vi "Extract Stage Status.vi"(11 "Table Stages":T4) -> (1 "Z Stage":T1, 2 "Y Stage":T1, 3 "X Stage":T1)   [LabVIEW 2018]
uses:
  Hardware Mfg/Thorlabs Translation Stages/Controls/Translation Stage Cluster.ctl
  Controls/Translation Stage Types.ctl
  Controls/Translation Stage Quick Status.ctl
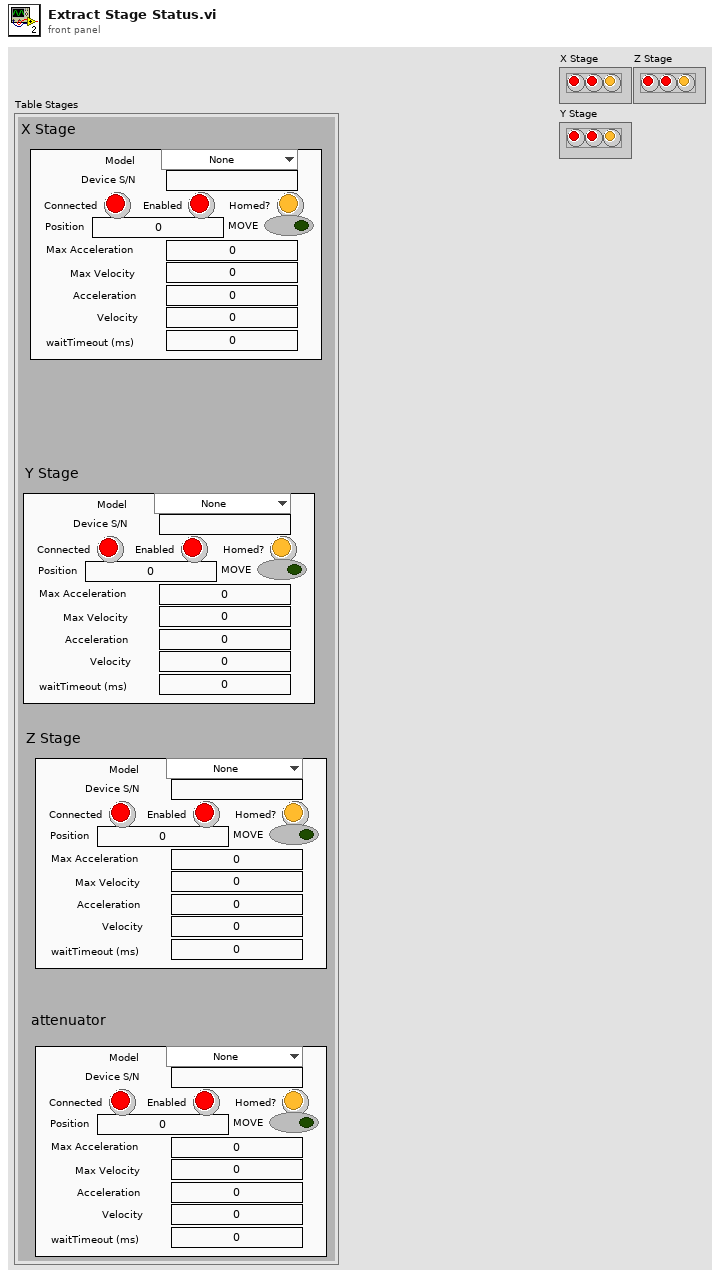
[diagram p1: front panel]
types:
  T1 = typedef "Translation Stage Quick Status.ctl" = cluster{"Is.Enabled?":bool, "Is.Connected?":bool, "Is.Homed?":bool}
  T2 = typedef "Translation Stage Cluster.ctl" = cluster{"Position":dbl, "Is.Enabled?":bool, "Is.Connected?":bool, "Device SN":string, "AccelerationMaximum":dbl, "VelocityMaximum":dbl, "Acceleration":dbl, "Velocity":dbl, "waitTimeout (ms)":i32, "Model":T3, "Is.Homed?":bool, "MOVE":bool}
  T3 = typedef "Translation Stage Types.ctl" = enum16{"None", "Thorlabs LTS", "Thorlabs MLJ"}
  T4 = cluster{"X Stage":T2, "Y Stage":T2, "Z Stage":T2, "attenuator":T2}
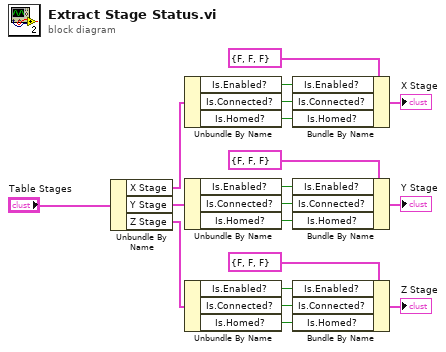
[diagram p0: block diagram]
diagram:
  n1 = Unbundle By Name("Table Stages") -> ("X Stage"=w16:T2, "Y Stage"=w15:T2, "Z Stage"=w14:T2)
  n2 = Unbundle By Name(w16) -> ("Is.Enabled?"=w9:bool, "Is.Connected?"=w8:bool, "Is.Homed?"=w7:bool)
  n3 = Unbundle By Name(w15) -> ("Is.Enabled?"=w6:bool, "Is.Connected?"=w5:bool, "Is.Homed?"=w4:bool)
  n4 = Unbundle By Name(w14) -> ("Is.Enabled?"=w3:bool, "Is.Connected?"=w2:bool, "Is.Homed?"=w1:bool)
  n5 = Bundle By Name(cluster=T1 {"Is.Enabled?"=FALSE, "Is.Connected?"=FALSE, "Is.Homed?"=FALSE} ("X Status"), "Is.Enabled?"=w9, "Is.Connected?"=w8, "Is.Homed?"=w7) -> (→"X Stage":T1)
  n6 = Bundle By Name(cluster=T1 {"Is.Enabled?"=FALSE, "Is.Connected?"=FALSE, "Is.Homed?"=FALSE} ("X Status"), "Is.Enabled?"=w6, "Is.Connected?"=w5, "Is.Homed?"=w4) -> (→"Y Stage":T1)
  n7 = Bundle By Name(cluster=T1 {"Is.Enabled?"=FALSE, "Is.Connected?"=FALSE, "Is.Homed?"=FALSE} ("X Status"), "Is.Enabled?"=w3, "Is.Connected?"=w2, "Is.Homed?"=w1) -> (→"Z Stage":T1)
